vi "unflattenFrequencyFromXML_Array.vi"(8 "error in (no error)":errorcluster, 9 "frequencyUnitInXML":T1, 10 "xmlString":string, 11 "frequencyForType":dbl[unit][](array[numeric])=[0.2617993877991494, 0.5235987755982988, 0.7853981633974482, 1.0471975511965976]) -> (0 "error out":errorcluster, 3 "frequency":dbl[unit][](array[numeric]))   [LabVIEW 2012, in "UnitsAndXML.lvlib"]
uses:
  <userlib>/Common/UnitsAndXML/UnitsAndXML.lvlib
  <userlib>/Common/UnitsAndXML/FlattenItemWithUnitToXML/FlattenFrequencyToXML/FrequencyUnit.ctl
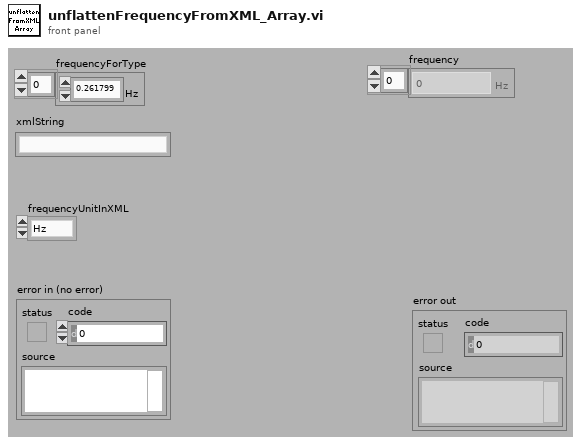
[diagram p1: front panel]
types:
  T1 = typedef "UnitsAndXML.lvlib/FrequencyUnit.ctl" = enum16{"Hz"}
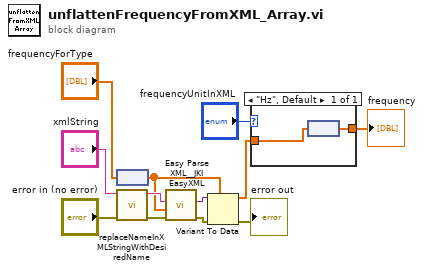
[diagram p0: block diagram]
diagram:
  n1 = node("frequencyForType") -> (w8:dbl[])
  n2 = call <userlib>:"replaceNameInXMLStringWithDesiredName.vi"("error in"="error in (no error)", "xmlString"="xmlString") -> ("error out"=w1:errorcluster, "revisedXMLString"=w9:string)  [unwired: 8 in]
  n3 = call <vilib>:"Easy Parse XML__JKI EasyXML.vi"("error in (no error)"=w1, "LabVIEW Data (Type)"=w8, "XML String"=w9) -> ("error out"=w4:errorcluster, "LabVIEW Data"=w11:variant)  [unwired: 7 in]
  n4 = Variant To Data(error in=w4, type=w8, Variant=w11) -> (data=w7:dbl[], error out=→"error out":errorcluster)
  n5 = case shown="\"Hz\", Default" "frequencyUnitInXML" {
    tunnel: w7 -> [w13]
    tunnel: [w14] -> w6
    frame "Hz", Default {
      n6 = node(w13) -> (w14:dbl[unit][])
    }
  }
  "frequency" <- w6
